vi "APS set trigger fifo data.vi"(6 "ShiftFlag":i32, 7 "ArraySize":i32, 8 "error in (no error)":errorcluster caption="错误输入（无错误）", 9 "DataArr":i32, 10 "FCmpCh":i32, 11 "Board_ID":i32) -> (0 "error out":errorcluster caption="错误输出", 1 "DataArr out":i32, 3 "function return":i32)   [LabVIEW 2011, in "APS168.lvlib"]
doc: "I32 FNTYPE APS_set_trigger_fifo_data( I32 Board_ID, I32 FCmpCh, I32 *DataArr, I32 ArraySize, I32 ShiftFlag );"
uses:
  APS168.lvlib
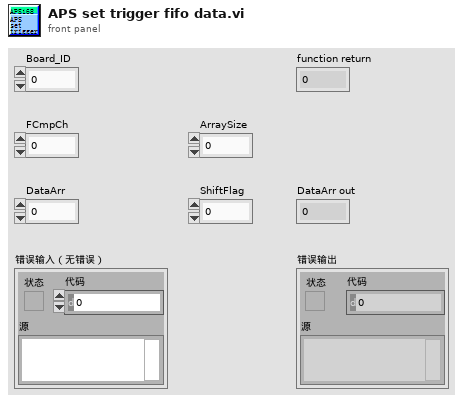
[diagram p1: front panel]
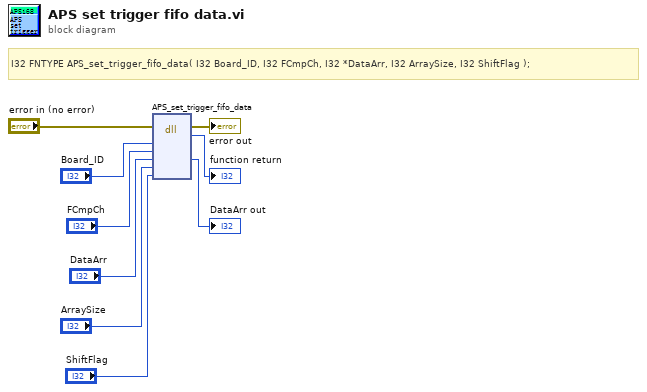
[diagram p0: block diagram]
diagram:
  # "I32 FNTYPE APS_set_trigger_fifo_data( I32 Board_ID, I32 FCmpCh, I32 *DataArr, I32 ArraySize, I32 ShiftFlag );"
  n1 = dll-call lib="PTH1Labs E软件ADLINK 204CAPS_1_7_1_LIB line 连续运动204APS168.*" fn="APS_set_trigger_fifo_data"(error in="error in (no error)", "Board_ID"="Board_ID", "FCmpCh"="FCmpCh", "DataArr"="DataArr", "ArraySize"="ArraySize", "ShiftFlag"="ShiftFlag") -> (error out=→"error out":errorcluster, →"function return":i32, "DataArr"=→"DataArr out":i32)  [unwired: 6 in, 1 out]
